vi "main.vi"() -> ()   [LabVIEW 2020]
panel:
  in  "file path":path
  in  "Boolean":bool
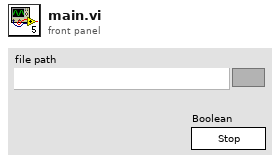
[diagram p1: front panel]
types:
  T1 = enum16{"open", "replace", "create", "open or create", "replace or create", "replace or create with confirmation"}
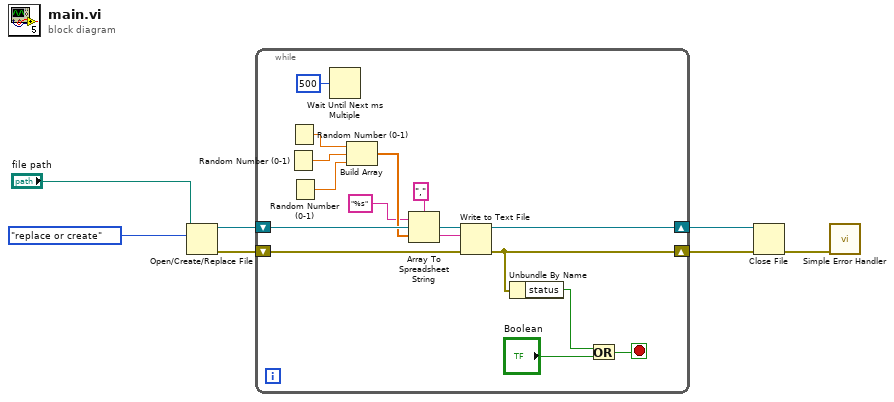
[diagram p0: block diagram]
diagram:
  n1 = Open/Create/Replace File(file path (use dialog)="file path", operation (0:open)=T1."replace or create") -> (refnum out=w7:refnum<file>, error out=w6:errorcluster)  [unwired: 4 in, 1 out]
  n2 = while {
    shift-right: [w16] -> w4
    shift-left: w6 -> [w18]
    shift-right: [w19] -> w5
    shift-left: w7 -> [w20]
    stop <- w17 stop-if-true
    n3 = Random Number (0-1)() -> (number: 0 to 1=w13:dbl)
    n4 = Random Number (0-1)() -> (number: 0 to 1=w14:dbl)
    n5 = Random Number (0-1)() -> (number: 0 to 1=w12:dbl)
    n6 = Wait Until Next ms Multiple(millisecond multiple=u32 500) -> ()  [unwired: 1 out]
    n7 = Build Array(w14, w13, w12) -> (w11:dbl[])
    n8 = Array To Spreadsheet String(delimiter (Tab)=",", array=w11, 3:"%s" ("format string")) -> (spreadsheet string=w10:string)
    n9 = Write to Text File(file (use dialog)=w20, text=w10, error in=w18) -> (refnum out=w19:refnum<file>, error out=w16:errorcluster)  [unwired: 1 in, 1 out]
    n10 = Unbundle By Name(w16) -> ("status"=w15:bool)
    n11 = Or(x=w15, y="Boolean") -> (x .or. y?=w17:bool)
  }
  n12 = Close File(refnum=w5, error in=w4) -> (error out=w3:errorcluster)  [unwired: 1 out]
  n13 = call <vilib>:"Simple Error Handler.vi"("error in (no error)"=w3) -> ()  [unwired: 4 in, 5 out]
